vi "ni579x Read EEPROM Device Data Header.vi"(0 "Register Bus":refnum<class "ni579x Register Bus v1 Host.lvclass">=refnum, 1 "scope":string(combo)="characterization data eeprom", 5 "start address":u32 format="%x", 11 "Error In":errorcluster) -> (4 "Register Bus (out)":refnum<class "ni579x Register Bus v1 Host.lvclass">, 6 "Device Data Header":T1={"Checksum"=0, "Number of Channels"=0, "Number of Attenuations"=[], "Number of Attenuator Settings"=[], "Number of Gain Settings"=[], "Pointer to Cal Data"=[], "Number of Reserved Bytes"=7, "Number of Frequencies"=[]} {"Checksum" format="%x"}, 15 "Error Out":errorcluster)   [LabVIEW 2013]
uses:
  <instrlib>/ni579x/Register Bus/v1/Host/ni579x Register Bus v1 Host.lvclass
  <instrlib>/ni579x/Config/v1/Shared/Types/EEPROM/ni579x EEPROM Device Data Header.ctl
  <instrlib>/ni579x/Config/v1/Shared/Conversions/From Byte Array (U8).vi
  <instrlib>/ni579x/Config/v1/Shared/Conversions/From Byte Array (U32).vi
  <instrlib>/ni579x/Config/v1/Shared/Conversions/From Byte Array (U16).vi
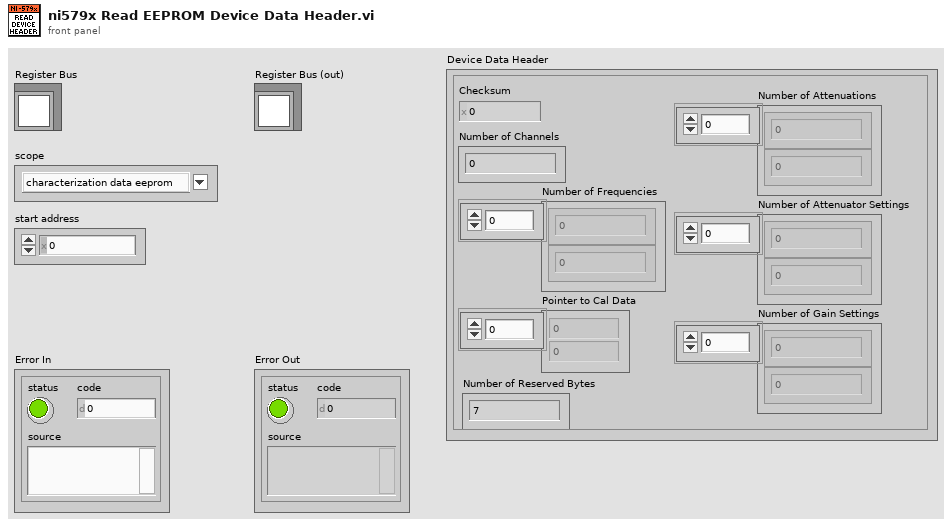
[diagram p1: front panel]
types:
  T1 = typedef "ni579x EEPROM Device Data Header.ctl" = cluster{"Checksum":u32, "Number of Channels":u8, "Number of Attenuations":u16[], "Number of Attenuator Settings":u8[], "Number of Gain Settings":u8[], "Pointer to Cal Data":u32[], "Number of Reserved Bytes":i32, "Number of Frequencies":u16[]}
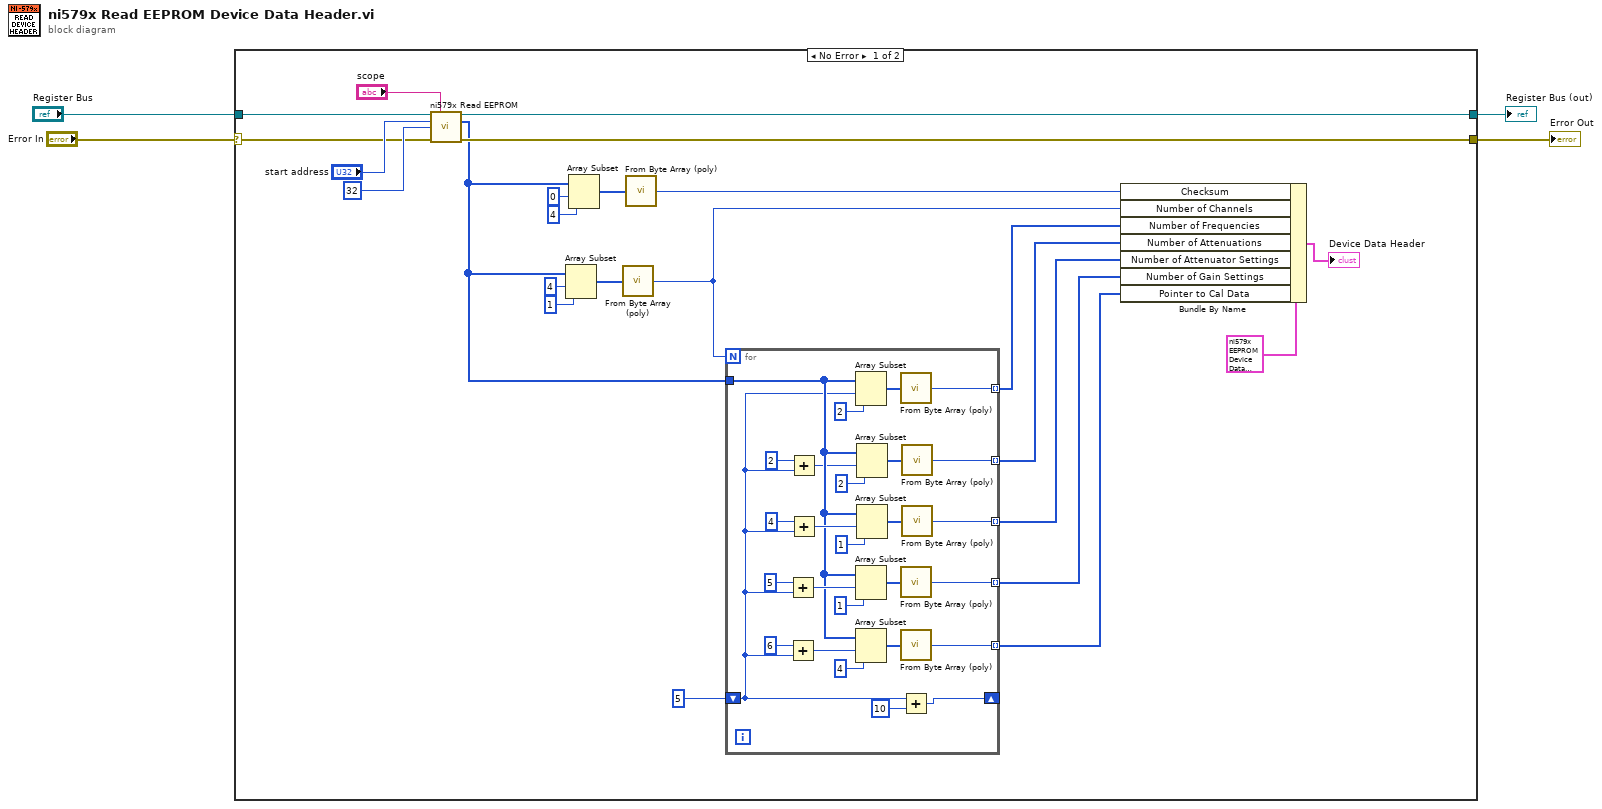
[diagram p0: block diagram]
diagram:
  n1 = case shown="No Error" "Error In" {
    selector: "Error In" -> [w25 w57]
    tunnel: [w16 w57] -> w3
    tunnel: "Register Bus" -> [w26 w56]
    tunnel: [w17 w56] -> w1
    frame No Error {
      n2 = call <instrlib>:"ni579x Read EEPROM.vi"("Register Bus"=w26, "scope"="scope", "start address"="start address", "size"=u32 32, "Error In"=w25) -> ("Register Bus (out)"=w17:refnum<class "ni579x Register Bus v1 Host.lvclass">, "data"=w13:u8[], "Error Out"=w16:errorcluster)  [unwired: 8 in]
      n3 = Array Subset(array=w13, index=4, length=1) -> (w20:u8[])
      n4 = Array Subset(array=w13, index=0, length=4) -> (w22:u8[])
      n5 = call-poly <instrlib>:"From Byte Array (poly).vi"("byte array in"=w20) -> ("element out"=w8:u8)
      n6 = call-poly <instrlib>:"From Byte Array (poly).vi"("byte array in"=w22) -> ("element out"=w21:u32)
      n7 = for {
        N: w8 -> [_]
        shift-right: [w36] -> _
        shift-left: 5 ("index") -> [w30]
        tunnel: w13 -> [w34]
        tunnel: [w53] -> w12 mode=indexing
        tunnel: [w40] -> w11 mode=indexing
        tunnel: [w39] -> w10 mode=indexing
        tunnel: [w38] -> w9 mode=indexing
        tunnel: [w29] -> w7 mode=indexing
        n8 = Add(x=5, y=w30) -> (x+y=w47:i32)
        n9 = Add(x=6, y=w30) -> (x+y=w42:i32)
        n10 = Add(x=2, y=w30) -> (x+y=w31:i32)
        n11 = Add(x=4, y=w30) -> (x+y=w50:i32)
        n12 = Array Subset(array=w34, index=w30, length=2) -> (w33:u8[])
        n13 = Array Subset(array=w34, index=w47, length=1) -> (w48:u8[])
        n14 = Array Subset(array=w34, index=w42, length=4) -> (w41:u8[])
        n15 = Array Subset(array=w34, index=w31, length=2) -> (w54:u8[])
        n16 = Array Subset(array=w34, index=w50, length=1) -> (w49:u8[])
        n17 = call-poly <instrlib>:"From Byte Array (poly).vi"("byte array in"=w33) -> ("element out"=w29:u16)
        n18 = call-poly <instrlib>:"From Byte Array (poly).vi"("byte array in"=w48) -> ("element out"=w39:u8)
        n19 = call-poly <instrlib>:"From Byte Array (poly).vi"("byte array in"=w41) -> ("element out"=w38:u32)
        n20 = Add(x=w30, y=10) -> (x+y=w36:i32)
        n21 = call-poly <instrlib>:"From Byte Array (poly).vi"("byte array in"=w54) -> ("element out"=w53:u16)
        n22 = call-poly <instrlib>:"From Byte Array (poly).vi"("byte array in"=w49) -> ("element out"=w40:u8)
      }
      n23 = Bundle By Name(cluster=T1 {"Checksum"=0, "Number of Channels"=2, "Number of Attenuations"=[255, 128], "Number of Attenuator Settings"=[2, 1], "Number of Gain Settings"=[64, 32], "Pointer to Cal Data"=[160, 68546], "Number of Reserved Bytes"=7, "Number of Frequencies"=[168, 168]} ("Device Data Header"), "Checksum"=w21, "Number of Channels"=w8, "Number of Frequencies"=w7, "Number of Attenuations"=w12, "Number of Attenuator Settings"=w11, "Number of Gain Settings"=w10, "Pointer to Cal Data"=w9) -> (→"Device Data Header":T1)
    }
    frame Error {
    }
  }
  "Register Bus (out)" <- w1
  "Error Out" <- w3
